vi "Supported Smart Syntax Representation.vi"(0 "String Operations in":refnum<class "String Functions.lvclass">, 11 "error in (no error)":errorcluster) -> (4 "String Operations out":refnum<class "String Functions.lvclass">, 6 "Smart Syntax Representation List":string[](array[string]), 15 "error out":errorcluster)   [LabVIEW 2019, in "String Functions.lvclass"]
uses:
  String Functions.lvclass
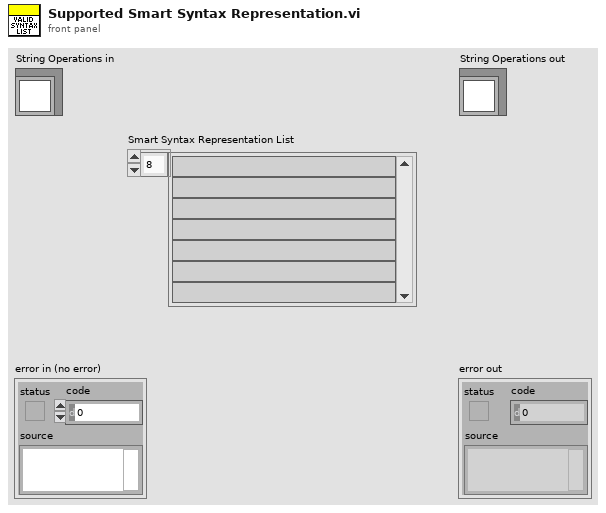
[diagram p1: front panel]
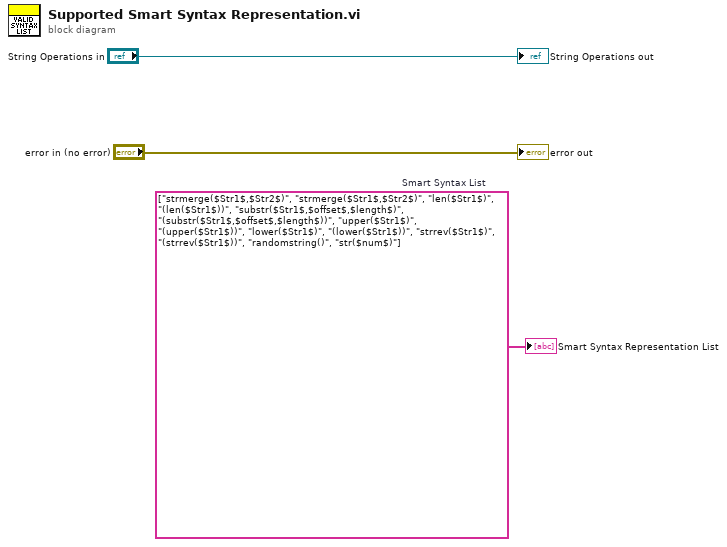
[diagram p0: block diagram]
diagram:
  w1 = string[] ["strmerge($Str1$,$Str2$)", "strmerge($Str1$,$Str2$)", "len($Str1$)", "(len($Str1$))", "substr($Str1$,$offset$,$length$)", "(substr($Str1$,$offset$,$length$))", "upper($Str1$)", "(upper($Str1$))", "lower($Str1$)", "(lower($Str1$))", "strrev($Str1$)", "(strrev($Str1$))", "randomstring()", "str($num$)"]  # Smart Syntax List
  "error out" <- "error in (no error)"
  "String Operations out" <- "String Operations in"
  "Smart Syntax Representation List" <- w1
